vi "Delaytime.vi"(7 "Density Value":u16, 8 "error in (no error)":errorcluster, 11 "Comport":refnum<visa-resource-name>) -> (0 "error out":errorcluster, 2 "Set Success":bool, 3 "Comport 2":refnum<visa-resource-name>)   [LabVIEW 2018]
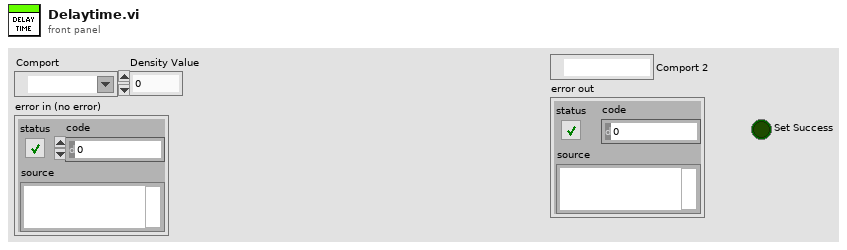
[diagram p1: front panel]
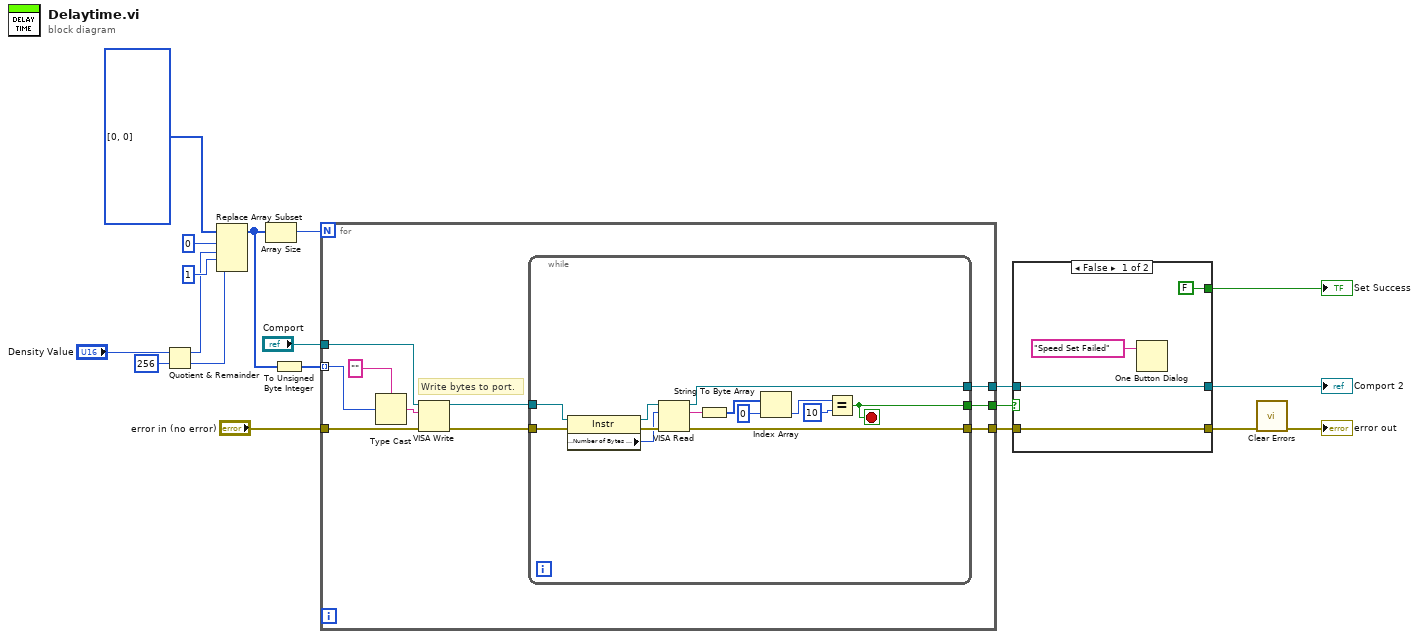
[diagram p0: block diagram]
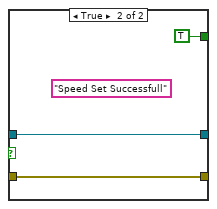
[diagram p2: hidden frame]
diagram:
  n1 = Quotient & Remainder(x="Density Value", y=u32 256) -> (x-y*floor(x/y)=w4:u32, floor(x/y)=w3:u32)
  n2 = Replace Array Subset(array=i16[] [0, 0], new element #1=w4, index #1=0 ("index"), new element #2=w3, index #2=1 ("index")) -> (w14:i16[])
  n3 = Array Size(array=w14) -> (size(s)=w8:i32)
  n4 = To Unsigned Byte Integer(number=w14) -> (unsigned 8bit integer=w2:u8[])
  n5 = for {
    N: w8 -> [_]
    tunnel: w2 -> [w24] mode=indexing
    tunnel: [w25] -> w9
    tunnel: [w23] -> w7
    tunnel: [w22] -> w6
    tunnel: "Comport" -> [w21]
    tunnel: "error in (no error)" -> [w20]
    # "Write bytes to port."
    n6 = Type Cast(type="", x=w24) -> (*(type *) &x=w28:string)
    n7 = VISA Write(VISA resource name=w21, write buffer=w28, error in (no error)=w20) -> (VISA resource name out=w27:refnum<visa-resource-name>, error out=w26:errorcluster)  [unwired: 1 out]
    n8 = while {
      tunnel: w27 -> [w34]
      tunnel: w26 -> [w33]
      tunnel: [w37] -> w25
      tunnel: [w36] -> w23
      tunnel: [w35] -> w22
      stop <- w37 stop-if-true
      n9 = property class="Instr"(reference=w34, error in=w33) -> (reference out=w32:refnum<visa-resource-name>, error out=w31:errorcluster, "Serial Settings:Number of Bytes at Serial Port"=w30:u32)
      n10 = VISA Read(VISA resource name=w32, byte count=w30, error in (no error)=w31) -> (VISA resource name out=w36:refnum<visa-resource-name>, read buffer=w42:string, error out=w35:errorcluster)  [unwired: 1 out]
      n11 = String To Byte Array(string=w42) -> (unsigned byte array=w41:u8[])
      n12 = Index Array(array=w41, index=0) -> (element=w39:u8)
      n13 = Equal?(x=w39, y=u8 10) -> (x = y?=w37:bool)
    }
  }
  n14 = case shown="False" w9 {
    tunnel: [FALSE TRUE] -> w10
    tunnel: w7 -> [w44 w48]
    tunnel: w6 -> [w43 w47]
    tunnel: [w44 w48] -> w18
    tunnel: [w43 w47] -> w17
    frame False {
      n15 = One Button Dialog(message="Speed Set Failed") -> ()  [unwired: 1 in, 1 out]
    }
    frame True {
      (unwired) "Speed Set Successfull" ("message")
    }
  }
  "Comport 2" <- w18
  "Set Success" <- w10
  n16 = call <vilib>:"Clear Errors.vi"("error in (no error)"=w17) -> ("error out"=→"error out":errorcluster)  [unwired: 5 in, 1 out]
